vi "Get Value.vi"(8 "error in (no error)":errorcluster, 11 "Ring Item Configuration in":refnum<class "Ring Item Configuration.lvclass">) -> (0 "error out":errorcluster, 2 "Project Info Value":string, 3 "Ring Item Configuration out":refnum<class "Ring Item Configuration.lvclass">)   [LabVIEW 2013, in "Item Configuration.lvlib" / "Ring Item Configuration.lvclass"]
uses:
  Ring Item Configuration.lvclass
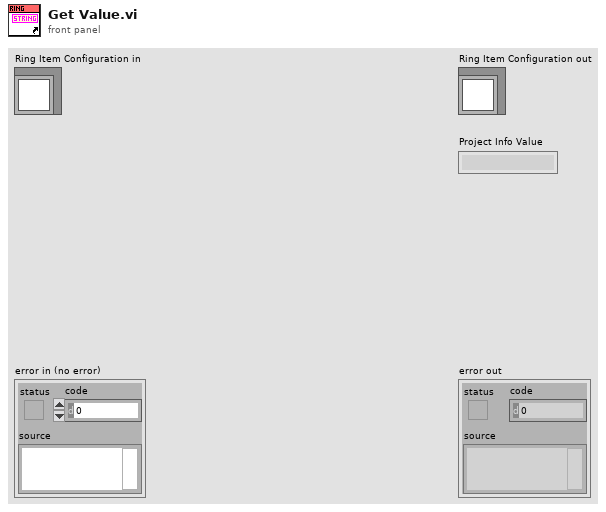
[diagram p1: front panel]
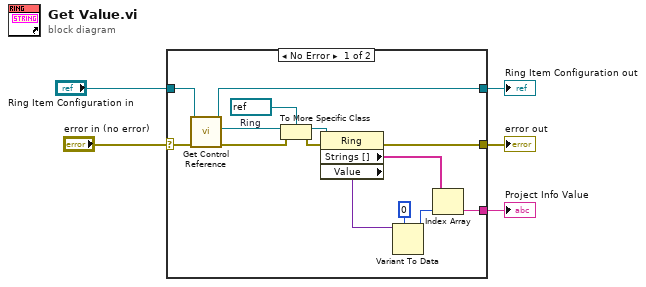
[diagram p0: block diagram]
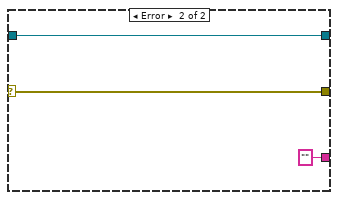
[diagram p2: hidden frame]
diagram:
  n1 = case shown="No Error" "error in (no error)" {
    selector: "error in (no error)" -> [w7 w22]
    tunnel: "Ring Item Configuration in" -> [w19 w20]
    tunnel: [w10 w22] -> w4
    tunnel: [w9 ""] -> w3
    tunnel: [w6 w20] -> w1
    frame No Error {
      w17 = refnum<vi> refnum  # Ring
      n2 = call-dynamic "Get Control Reference.vi"("error in (no error)"=w7, "Item Configuration in"=w19) -> ("error out"=w16:errorcluster, "Control Reference"=w18:refnum<vi>, "Item Configuration out"=w6:refnum<class "Ring Item Configuration.lvclass">)  [unwired: 7 in]
      n3 = To More Specific Class(target class=w17, reference=w18, error in=w16) -> (specific class reference=w14:refnum<vi>, error out=w15:errorcluster)
      n4 = property class="Ring"(reference=w14, error in=w15) -> (error out=w10:errorcluster, "Strings []"=w8:string[], "Value"=w11:variant)  [unwired: 1 out]
      n5 = Variant To Data(type=0 ("index"), Variant=w11) -> (data=w12:i32)  [unwired: 1 in, 1 out]
      n6 = Index Array(array=w8, index=w12) -> (element=w9:string)
    }
    frame Error {
    }
  }
  "error out" <- w4
  "Ring Item Configuration out" <- w1
  "Project Info Value" <- w3
